vi "SDF Small Gasifierl HMI - Alarm Display Page.vi"() -> ()   [LabVIEW 2013]
uses:
  <vilib>/NI/Current Value Table/DataTypes/Boolean_Write.vi
  <vilib>/NI/Current Value Table/DataTypes/Double_Write.vi
  <vilib>/NI/Current Value Table/DataTypes/Boolean_Read.vi
  <vilib>/NI/Current Value Table/DataTypes/Double_Read.vi
  <vilib>/NI/Current Value Table/Type to Enum.vi
  <vilib>/NI/Current Value Table/DataTypes/Boolean_Type To Enum.vi
  <vilib>/NI/Current Value Table/DataTypes/Double_Type To Enum.vi
  <vilib>/NI/Current Value Table/FGVs/CVT Globals.vi
  <vilib>/NI/Current Value Table/FGVs/Tag Memory.vi
  <vilib>/NI/Current Value Table/Memory Block.vi
  <vilib>/NI/Current Value Table/DataTypes/Boolean_Memory Block.vi
  <vilib>/NI/Current Value Table/DataTypes/Double_Memory Block.vi
  <vilib>/NI/Current Value Table/Current Value Table.lvlib
panel:
  in  "Clear":bool
  in  "Numeric":dbl
  out "TI-101":bool
  out "TI-101":dbl
  in  "To Back":bool caption="Caption"
  in  "To CVT Viewer":bool caption="Caption"
  in  "Stop":bool caption="Caption"
  in  "To Machine Control":bool caption="Caption"
  out "Page's Title":string="Manual Control"
  # "Home"
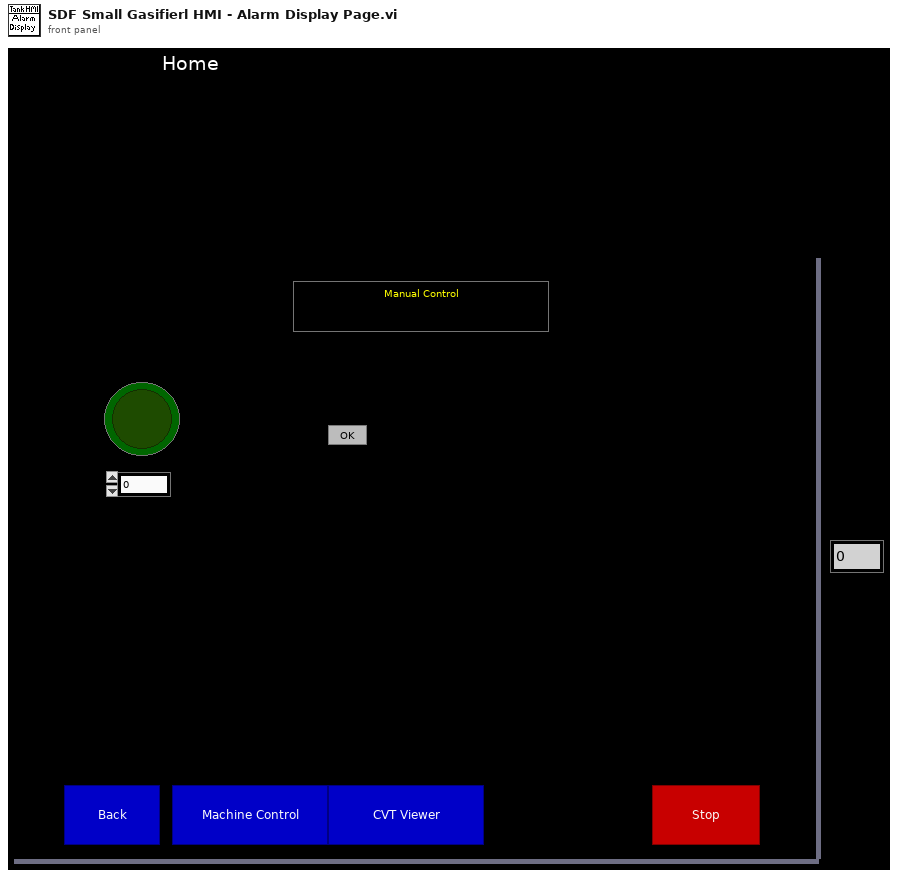
[diagram p1: front panel]
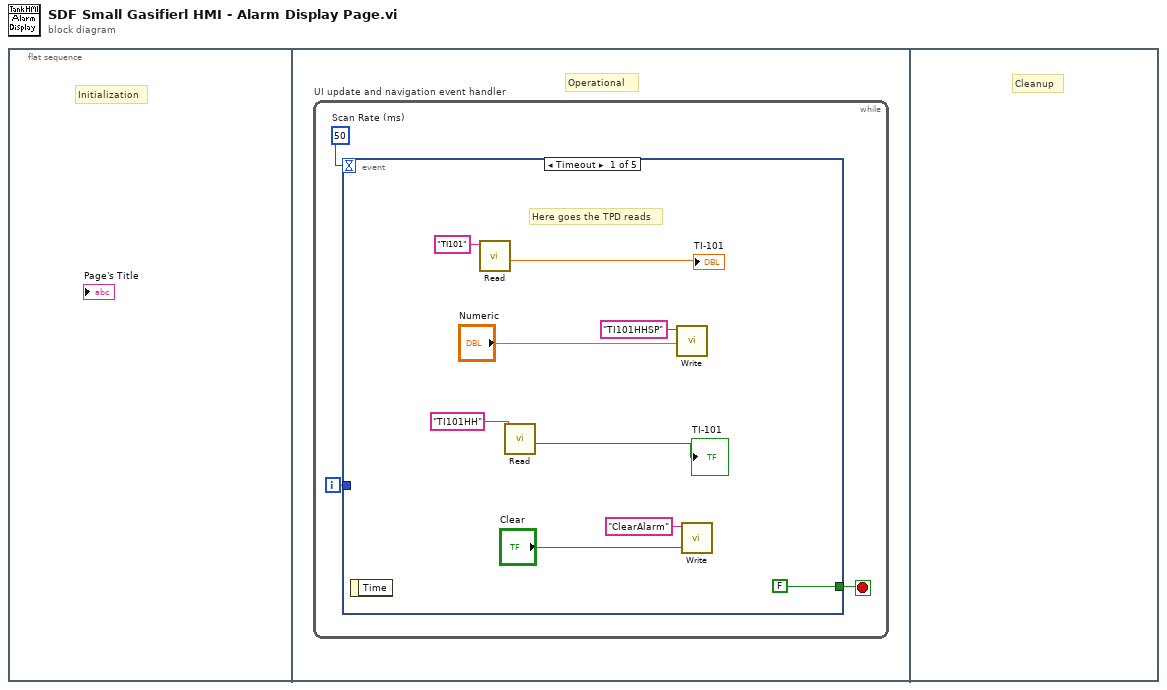
[diagram p0: block diagram]
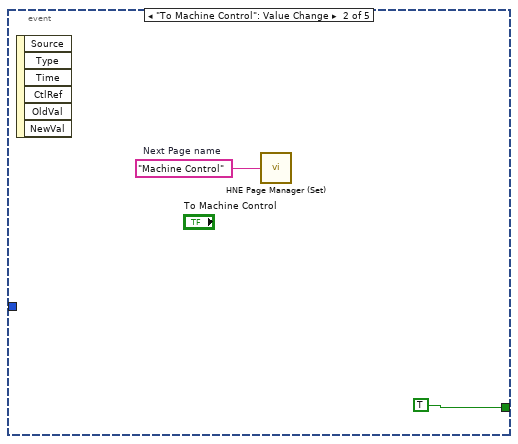
[diagram p2: hidden frame]
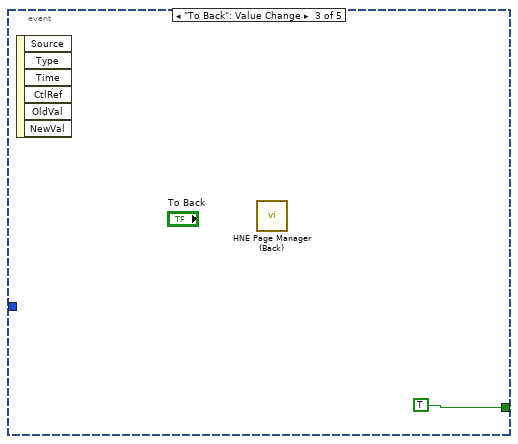
[diagram p3: hidden frame]
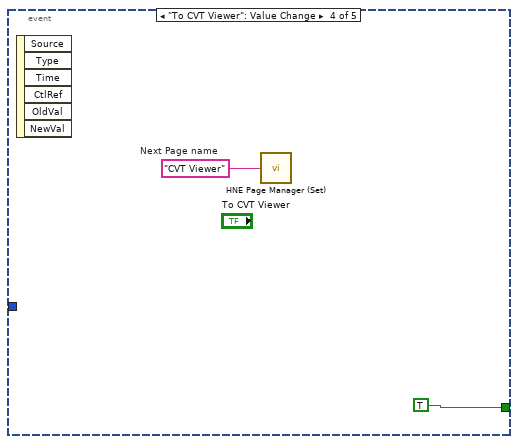
[diagram p4: hidden frame]
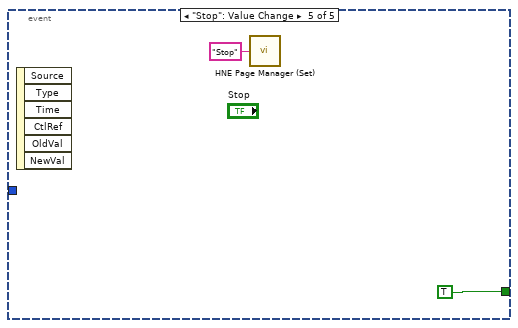
[diagram p5: hidden frame]
diagram:
  n1 = flat-sequence {
    frame #0 {
      # "Initialization"
    }
    frame #1 {
      # "Operational"
      n2 = while "UI update and navigation event handler" {
        i -> [w2]
        stop <- w3 stop-if-true
        w1 = 50  # Scan Rate (ms)
        n3 = event shown="[0] Timeout" {
          selector: _ -> [_ _ _ _ _]
          dyn-events: _ -> [_ _ _ _ _]
          timeout: w1 -> [_ _ _ _ _]
          tunnel: [FALSE ("Page Name") TRUE ("Page Name") TRUE ("Page Name") TRUE ("Page Name") TRUE ("Page Name")] -> w3
          tunnel: w2 -> [_ _ _ _ _]
          event Timeout {
            # "Here goes the TPD reads"
            n4 = event-data() -> ()  [unwired: 1 in, 1 out]
            n5 = call-poly <vilib>:"Read.vi"("Tag Name"="TI101") -> ("Value"=→"TI-101":dbl)  [unwired: 9 in, 1 out]
            n6 = call-poly <vilib>:"Read.vi"("Tag Name"="TI101HH") -> ("Value"=→"TI-101":bool)  [unwired: 9 in, 1 out]
            n7 = call-poly <vilib>:"Write.vi"("Value"="Numeric", "Tag Name"="TI101HHSP") -> ()  [unwired: 9 in, 1 out]
            n8 = call-poly <vilib>:"Write.vi"("Value"="Clear", "Tag Name"="ClearAlarm") -> ()  [unwired: 9 in, 1 out]
          }
          event "To Machine Control": Value Change {
            w14 = "Machine Control"  # Next Page name
            n9 = event-data() -> ()  [unwired: 1 in, 6 out]
            n10 = call <userlib>:"HNE Page Manager (Set).vi"("Next Page"=w14) -> ()  [unwired: 4 in, 1 out]
          }
          event "To Back": Value Change {
            n11 = event-data() -> ()  [unwired: 1 in, 6 out]
            n12 = call <userlib>:"HNE Page Manager (Back).vi"() -> ()  [unwired: 5 in, 1 out]
          }
          event "To CVT Viewer": Value Change {
            w17 = "CVT Viewer"  # Next Page name
            n13 = event-data() -> ()  [unwired: 1 in, 6 out]
            n14 = call <userlib>:"HNE Page Manager (Set).vi"("Next Page"=w17) -> ()  [unwired: 4 in, 1 out]
          }
          event "Stop": Value Change {
            n15 = event-data() -> ()  [unwired: 1 in, 6 out]
            n16 = call <userlib>:"HNE Page Manager (Set).vi"("Next Page"="Stop") -> ()  [unwired: 4 in, 1 out]
          }
        }
      }
    }
    frame #2 {
      # "Cleanup"
    }
  }
